vi "convert excel to xml encoding (ni-aim).vi"(11 "excel encoding":T1) -> (3 "xml encoding":i32)   [LabVIEW 2020]
uses:
  Controls/Encoding.ctl
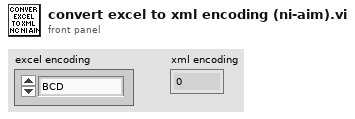
[diagram p1: front panel]
types:
  T1 = typedef "Encoding.ctl" = enum16{"BCD", "BNR", "Discrete"}
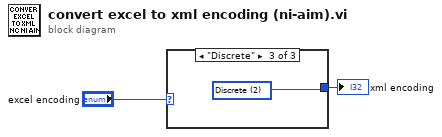
[diagram p0: block diagram]
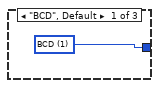
[diagram p2: hidden frame]
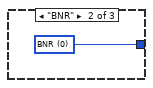
[diagram p3: hidden frame]
diagram:
  n1 = case shown="\"Discrete\"" "excel encoding" {
    tunnel: [w3 w4 w5] -> w1
    frame "BCD", Default {
      w3 = 1 items=["BNR", "BCD", "Discrete"] ("encoding")
    }
    frame "BNR" {
      w4 = 0 items=["BNR", "BCD", "Discrete"] ("encoding")
    }
    frame "Discrete" {
      w5 = 2 items=["BNR", "BCD", "Discrete"] ("encoding")
    }
  }
  "xml encoding" <- w1
